vi "Sequence by Name.vi"(8 "error in (no error)":errorcluster, 10 "Sequence Name":string, 11 "SequenceFile in":refnum<class "SequenceFile.lvclass">) -> (0 "error out":errorcluster, 2 "Sequence":refnum<class "Sequence.lvclass">, 3 "SequenceFile out":refnum<class "SequenceFile.lvclass">)   [LabVIEW 2020, in "TSnax.lvlib" / "SequenceFile.lvclass"]
uses:
  SequenceFile.lvclass
  SequenceFile.lvclass/SequenceFile.ctl
  Sequence/Sequence.lvclass
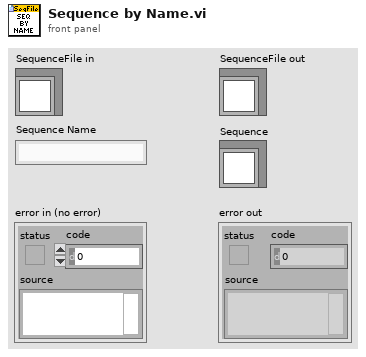
[diagram p1: front panel]
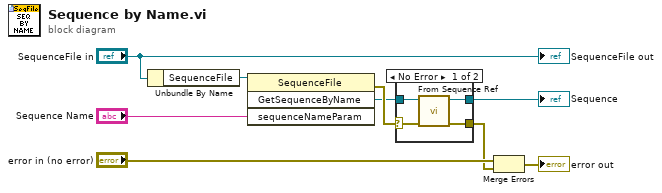
[diagram p0: block diagram]
diagram:
  n1 = Unbundle By Name("SequenceFile in") -> ("SequenceFile"=w6:refnum<k7>)
  n2 = invoke class="SequenceFile" method="GetSequenceByName"(reference=w6, "sequenceNameParam"="Sequence Name") -> (error out=w9:errorcluster, "GetSequenceByName"=w4:refnum<k7>)  [unwired: 2 in, 2 out]
  n3 = case shown="No Error" w9 {
    selector: w9 -> [w13 w14]
    tunnel: w4 -> [w12 _]
    tunnel: [w11 _] -> w3
    tunnel: [w10 w14] -> w1
    frame No Error {
      n4 = call "From Sequence Ref.vi"("error in (no error)"=w13, "Sequence"=w12) -> ("error out"=w10:errorcluster, "Sequence out"=w11:refnum<class "Sequence.lvclass">)  [unwired: 8 in]
    }
    frame Error {
    }
  }
  "Sequence" <- w3
  n5 = Merge Errors("error in (no error)", w1) -> (→"error out":errorcluster)
  "SequenceFile out" <- "SequenceFile in"
